vi "Define Parameter.vi"(8 "error in (no error)":errorcluster, 11 "Analyze BaseClass in":refnum<class "Analyze BaseClass.lvclass">) -> (0 "error out":errorcluster, 3 "Analyze BaseClass out":refnum<class "Analyze BaseClass.lvclass">)   [LabVIEW 2020, in "Analyze.lvlib" / "Analyze BaseClass.lvlib" / "Analyze BaseClass.lvclass"]
uses:
  Analyze BaseClass.lvclass
  Analyze Parameter/Analyze Parameter ROI/Analyze Parameter ROI.lvclass
  C:/POLARIS Programme/POLARIS-AS-3-Cams/Submodules/HIJ Vision/Analyze/Analyze Parameter/Analyze Parameter Base/Analyze Parameter Base.lvclass
  Analyze Parameter/Analyze Parameter Calibration/Analyze Parameter Calibration.lvclass
  Analyze BaseClass.lvclass/Analyze BaseClass.ctl
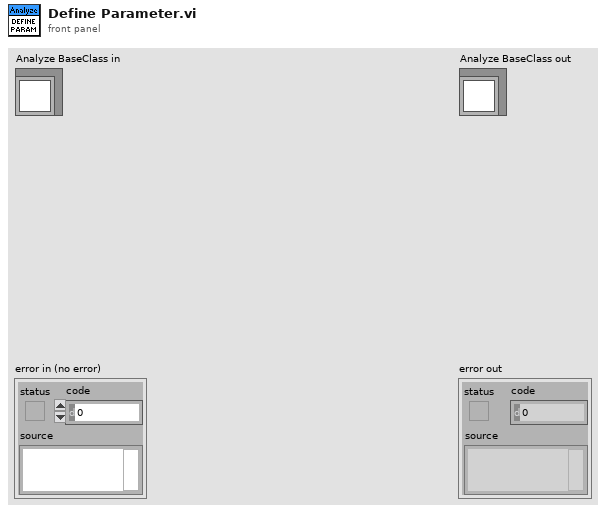
[diagram p1: front panel]
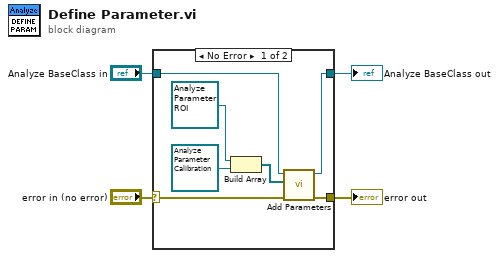
[diagram p0: block diagram]
diagram:
  n1 = case shown="No Error" "error in (no error)" {
    selector: "error in (no error)" -> [w9 w13]
    tunnel: [w8 w13] -> w3
    tunnel: [w10 w12] -> w1
    tunnel: "Analyze BaseClass in" -> [w11 w12]
    frame No Error {
      n2 = Build Array(refnum<class "Analyze Parameter ROI.lvclass"> refnum ("Analyze Parameter ROI.lvclass"), refnum<class "Analyze Parameter Calibration.lvclass"> refnum ("Analyze Parameter Calibration.lvclass")) -> (w5:refnum<class "Analyze Parameter Base.lvclass">[])
      n3 = call-dynamic "Add Parameters.vi"("error in (no error)"=w9, "Parameters"=w5, "Analyze BaseClass in"=w11) -> ("error out"=w8:errorcluster, "Analyze BaseClass out"=w10:refnum<class "Analyze BaseClass.lvclass">)  [unwired: 7 in]
    }
    frame Error {
    }
  }
  "error out" <- w3
  "Analyze BaseClass out" <- w1
